vi "Set Server State.vi"(8 "error in":errorcluster, 10 "New State":T1, 11 "gRPC server in":refnum<class "Servicer.lvclass">) -> (0 "error out":errorcluster, 2 "Previous State":T1, 3 "gRPC server out":refnum<class "Servicer.lvclass">)   [LabVIEW 2019, in "gRPC-servicer.lvlib" / "Servicer.lvclass"]
uses:
  Servicer.lvclass
  typeDefs/Server State Data.ctl
  Servicer.lvclass/Servicer.ctl
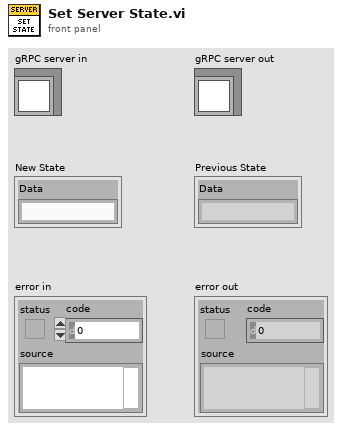
[diagram p1: front panel]
types:
  T1 = typedef "gRPC-servicer.lvlib/Servicer.lvclass/Server State Data.ctl" = cluster{"Data":string}
  T2 = typedef "Template Server.lvlib/Template Server.lvclass/Server State Data.ctl" = cluster{"Data":string}
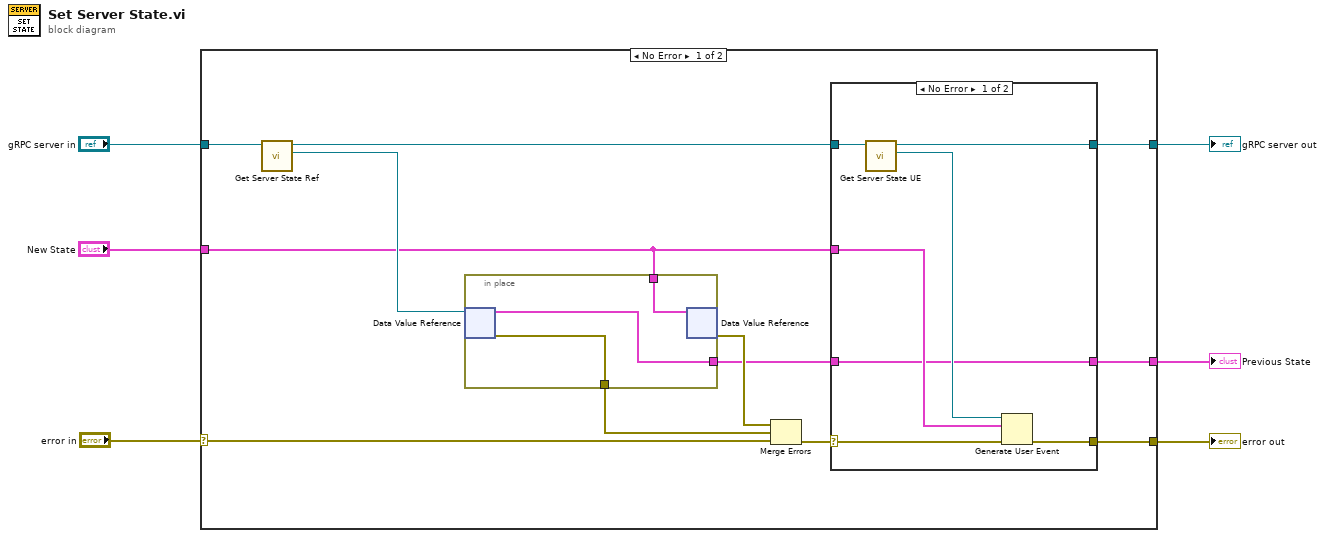
[diagram p0: block diagram]
diagram:
  n1 = case shown="No Error" "error in" {
    selector: "error in" -> [w18 w33]
    tunnel: [w14 w33] -> w5
    tunnel: [w10 w32] -> w3
    tunnel: "gRPC server in" -> [w13 w32]
    tunnel: "New State" -> [w9 _]
    tunnel: [w7 _] -> w1
    frame No Error {
      n2 = call "Get Server State Ref.vi"("gRPC server in"=w13) -> ("Server State Ref"=w12:refnum<data-value>, "gRPC server out"=w11:refnum<class "Servicer.lvclass">)  [unwired: 9 in]
      n3 = in-place {
        in-place-border: w9 -> [w30]
        in-place-border: [w29] -> w8
        in-place-border: [w31] -> w17
        n4 = in-place-dvr #1(w12) -> (w29:T2, w31:errorcluster)
        n5 = in-place-dvr #1(w30) -> (w16:errorcluster)  [unwired: 1 out]
      }
      n6 = Merge Errors(w16, w17, w18) -> (w15:errorcluster)
      n7 = case shown="No Error" w15 {
        selector: w15 -> [w25 w28]
        tunnel: w11 -> [w23 w27]
        tunnel: [w24 w28] -> w14
        tunnel: [w22 w27] -> w10
        tunnel: w9 -> [w20 _]
        tunnel: w8 -> [w19 w26]
        tunnel: [w19 w26] -> w7
        frame No Error {
          n8 = call "Get Server State UE.vi"("gRPC server in"=w23) -> ("Server Internal State UE"=w21:refnum<user-event>, "gRPC server out"=w22:refnum<class "Servicer.lvclass">)  [unwired: 9 in]
          n9 = Generate User Event(user event=w21, event data cluster=w20, error in=w25) -> (error out=w24:errorcluster)  [unwired: 1 in, 1 out]
        }
        frame Error {
        }
      }
    }
    frame Error {
    }
  }
  "error out" <- w5
  "gRPC server out" <- w3
  "Previous State" <- w1
